vi "finish_photon_stream.vi"(8 "error in (no error)":errorcluster, 11 "tt20 in":refnum<class "tt20.lvclass">) -> (0 "error out":errorcluster, 3 "tt20 out":refnum<class "tt20.lvclass">)   [LabVIEW 2015, in "tt20.lvclass"]
uses:
  tt20.lvclass
  tt20.lvclass/tt20.ctl
  C:/Users/MX-Microscope/Documents/LabVIEW Data/lvoop_campus_2018/Detector_Class/Swabian/time_tagger_vis/TTCSharp32.dll
  time_tagger_vis/TTCSharp32.dll
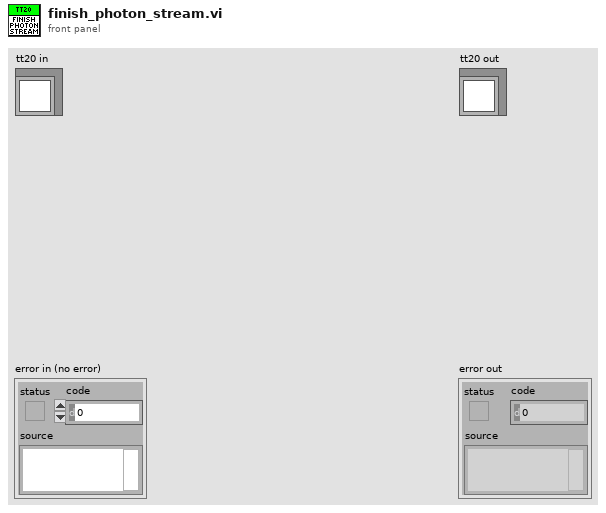
[diagram p1: front panel]
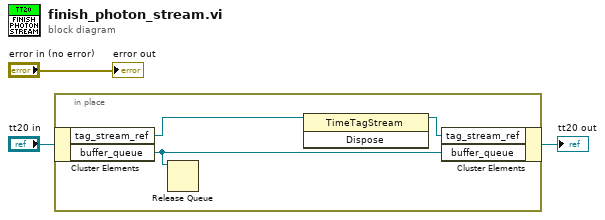
[diagram p0: block diagram]
diagram:
  n1 = in-place {
    n2 = in-place-cluster #1("tt20 in") -> ("tag_stream_ref"=w4:refnum<k24>, "buffer_queue"=w5:refnum<queue>)
    n3 = Release Queue(queue=w5) -> ()  [unwired: 2 in, 3 out]
    n4 = invoke class="TimeTagStream" method="Dispose"(reference=w4) -> (reference out=w6:refnum<k24>)  [unwired: 2 in, 2 out]
    n5 = in-place-cluster #1("tag_stream_ref"=w6, "buffer_queue"=w5) -> (→"tt20 out":refnum<class "tt20.lvclass">)
  }
  "error out" <- "error in (no error)"
